vi "Water_Level_control_PID.vi"() -> ()   [LabVIEW 2026]
uses:
  <vilib>/addons/control/pid/pid.llb/PID (DBL).vi
  <vilib>/addons/control/pid/NI_PID_pid.lvlib
panel:
  in  "stop":bool
  in  "Kd":dbl=0.01
  in  "Ki":dbl=0.5
  in  "Kp":dbl=0.3
  out "Current Level":dbl=-52.583284554687495
  out "Current Flow":dbl=-100.0
  out "Actual Liquid Level":dbl(slide)=-52.583284554687495 scale=0.0..10.0
  in  "Desired Liquid Level (m)":dbl=5.0
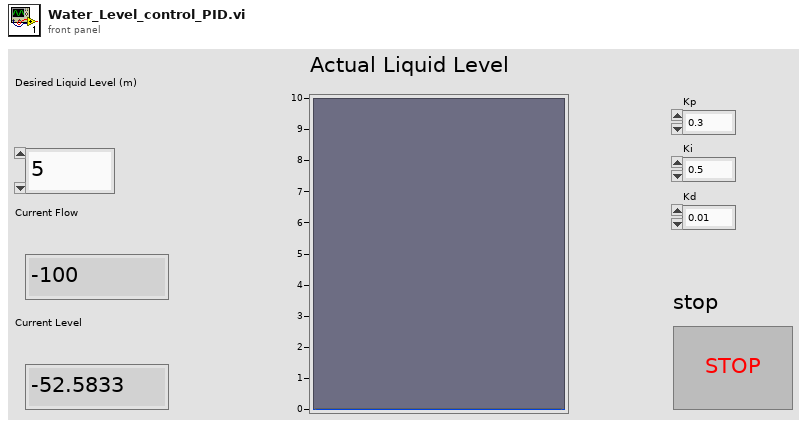
[diagram p1: front panel]
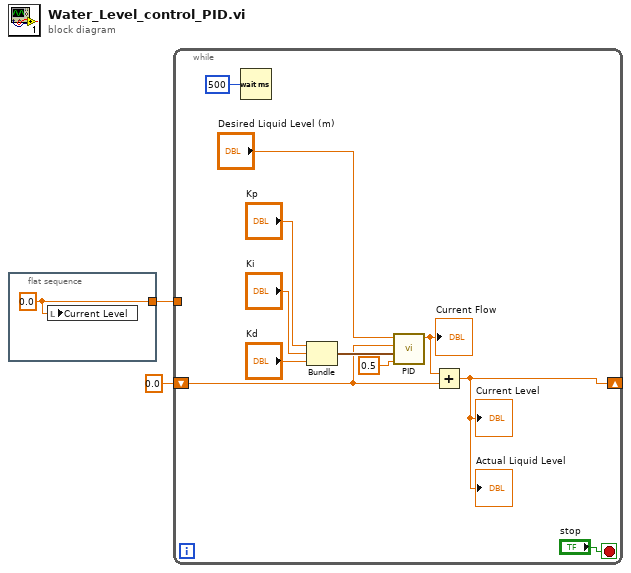
[diagram p0: block diagram]
diagram:
  n1 = flat-sequence {
    tunnel: [w3] -> w1
    frame #0 {
      w3 = 0.0 ("Current Level")
      n2 = local write "Current Level"(w3) -> ()
    }
  }
  n3 = while {
    shift-right: [w4] -> _
    shift-left: 0.0 -> [w5]
    tunnel: w1 -> [_]
    stop <- "stop" stop-if-true
    n4 = Wait (ms)(milliseconds to wait=500) -> ()  [unwired: 1 out]
    n5 = Bundle("Kp"="Kp", "Ki"="Ki", "Kd"="Kd") -> (w8:cluster{"Kp":dbl, "Ki":dbl, "Kd":dbl})  [unwired: 1 in]
    n6 = call-poly <vilib>:"PID.vi"("dt (s)"=0.5, "PID gains"=w8, "process variable"=w5, "setpoint"="Desired Liquid Level (m)") -> ("output"=w6:dbl)  [unwired: 6 in, 1 out]
    "Current Flow" <- w6
    n7 = Add(x=w6, y=w5) -> (x+y=w4:dbl)
    "Actual Liquid Level" <- w4
    "Current Level" <- w4
  }
